vi "Read Address_modified.vi"(0 "VISA resource name":refnum<visa-resource-name>, 5 "Motor ID (0)":u8, 7 "Address number (0)":u8 max=49, 9 "Number of Addresses to read (1)":u8=1, 11 "Error in (no error)":errorcluster) -> (4 "VISA resource name Out":refnum<visa-resource-name>, 6 "Data Read":u8[](array[numeric]), 10 "Motor Error Status":T1, 15 "error out":errorcluster)   [LabVIEW 2015, in "Dynamixel Motor.lvlib"]
doc: "Reads an arbitrary number of consecutive addresses from a motor's register. This is a Low-Level VI that is used by other VIs."
uses:
  <instrlib>/Dynamixel Motor/Public/Motor Operation/Low Level/Alarm Setting.ctl
  <instrlib>/Dynamixel Motor/Dynamixel Motor.lvlib
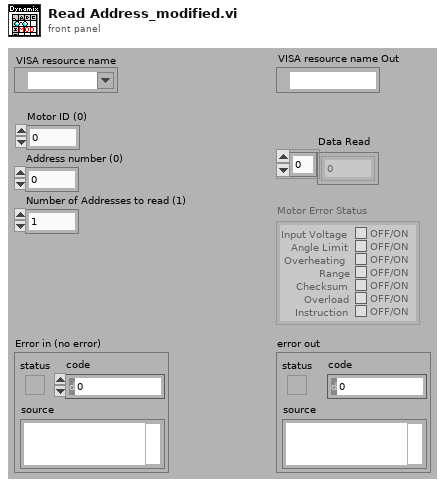
[diagram p1: front panel]
types:
  T1 = typedef "Dynamixel Motor.lvlib/Alarm Setting.ctl" = cluster{"Input Voltage":bool, "Angle Limit":bool, "Overheating ":bool, "Range":bool, "Checksum":bool, "Overload":bool, "Instruction":bool}
  T2 = cluster{"Boolean array[0]":bool, "Boolean array[1]":bool, "Boolean array[2]":bool, "Boolean array[3]":bool, "Boolean array[4]":bool, "Boolean array[5]":bool, "Boolean array[6]":bool}
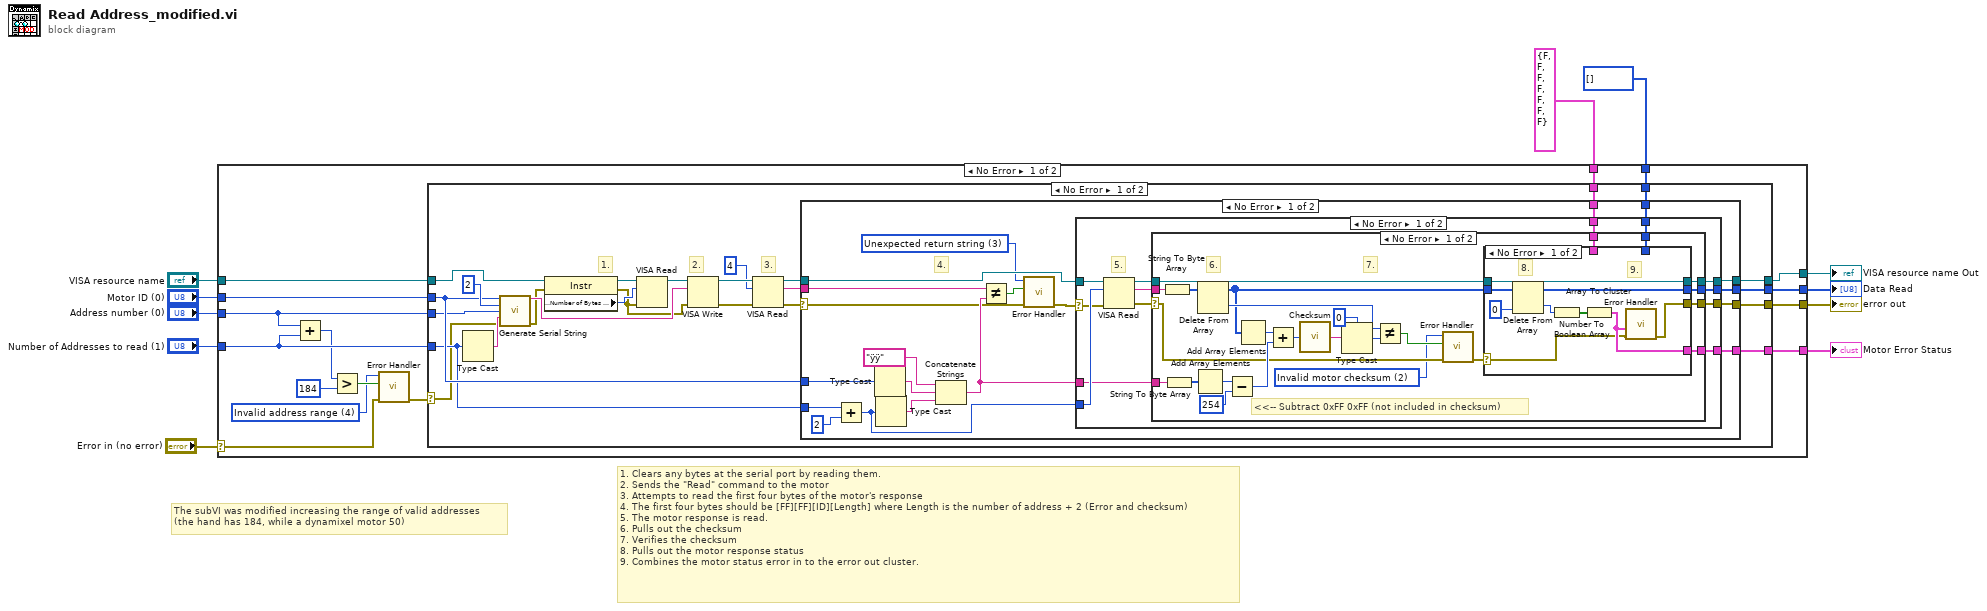
[diagram p0: block diagram]
diagram:
  # "The subVI was modified increasing the range of valid addresses\n(the hand has 184, while a dynamixel motor 50)"
  # "1. Clears any bytes at the serial port by reading them.\n2. Sends the \"Read\" command to the motor\n3. Attempts to read the first four bytes of the motor's response\n4. The first four bytes should be [FF][FF][ID][Length] where Length is the number of address + 2 (Error and checksum)\n5. The motor response is read.\n6. Pulls out the checksum\n7. Verifies the checksum\n8. Pulls out the motor response status\n9. Combines the motor status error in to the error out cluster."
  n1 = case shown="No Error" "Error in (no error)" {
    selector: "Error in (no error)" -> [w16 w143]
    tunnel: "Address number (0)" -> [w20 _]
    tunnel: [w23 w141] -> w10
    tunnel: "VISA resource name" -> [w27 w142]
    tunnel: "Number of Addresses to read (1)" -> [w21 _]
    tunnel: "Motor ID (0)" -> [w25 _]
    tunnel: [w26 w142] -> w6
    tunnel: [w24 w143] -> w5
    tunnel: [w22 w140] -> w3
    tunnel: u8[] [] ("unsigned byte array") -> [w14 w141]
    tunnel: T2 {"Boolean array[0]"=FALSE, "Boolean array[1]"=FALSE, "Boolean array[2]"=FALSE, "Boolean array[3]"=FALSE, "Boolean array[4]"=FALSE, "Boolean array[5]"=FALSE, "Boolean array[6]"=FALSE} ("Boolean array") -> [w13 w140]
    frame No Error {
      w12 = u16 4 items=["Scan timeout"=1, "Invalid motor checksum"=2, "Unexpected return string"=3, "Invalid address range"=4] ("Error type")
      n2 = Add(x=w20, y=w21) -> (x+y=w19:u8)
      n3 = Greater?(x=w19, y=u8 184) -> (0:w15:bool)
      n4 = call <instrlib>:"Error Handler.vi"("error in (no error)"=w16, "Error? (no error)"=w15, "Error type"=w12) -> ("error out"=w17:errorcluster)  [unwired: 8 in]
      n5 = case shown="No Error" w17 {
        selector: w17 -> [w30 w138]
        tunnel: w27 -> [w49 w139]
        tunnel: [w48 w139] -> w26
        tunnel: w25 -> [w42 _]
        tunnel: [w40 w138] -> w24
        tunnel: [w39 w137] -> w23
        tunnel: [w38 w136] -> w22
        tunnel: w21 -> [w32 _]
        tunnel: w20 -> [w31 _]
        tunnel: w14 -> [w29 w137]
        tunnel: w13 -> [w28 w136]
        frame No Error {
          # "3."
          # "2."
          # "1."
          n6 = Type Cast(x=w32) -> (*(type *) &x=w33:string)  [unwired: 1 in]
          n7 = call <instrlib>:"Generate Serial String.vi"("Motor ID"=w42, "Command"=u8 2, "Address"=w31, "Parameters"=w33, "Error in (no error)"=w30) -> ("Command to Serial"=w50:string, "error out"=w45:errorcluster)  [unwired: 9 in]
          n8 = property class="Instr"(reference=w49, error in=w45) -> (reference out=w46:refnum<visa-resource-name>, error out=w41:errorcluster, "Serial Settings:Number of Bytes at Serial Port"=w47:u32)
          n9 = VISA Read(VISA resource name=w46, byte count=w47, error in (no error)=w41) -> (VISA resource name out=w52:refnum<visa-resource-name>)  [unwired: 3 out]
          n10 = VISA Write(VISA resource name=w52, write buffer=w50, error in (no error)=w41) -> (VISA resource name out=w51:refnum<visa-resource-name>, error out=w44:errorcluster)  [unwired: 1 out]
          n11 = VISA Read(VISA resource name=w51, byte count=u32 4, error in (no error)=w44) -> (VISA resource name out=w34:refnum<visa-resource-name>, read buffer=w37:string, error out=w35:errorcluster)  [unwired: 1 out]
          n12 = case shown="No Error" w35 {
            selector: w35 -> [w58 w135]
            tunnel: w32 -> [w71 _]
            tunnel: w42 -> [w70 _]
            tunnel: w37 -> [w57 _]
            tunnel: [w64 w135] -> w40
            tunnel: w34 -> [w66 w134]
            tunnel: [w65 w134] -> w48
            tunnel: [w61 w133] -> w39
            tunnel: [w60 w132] -> w38
            tunnel: w29 -> [w55 w133]
            tunnel: w28 -> [w54 w132]
            frame No Error {
              w53 = u16 3 items=["Scan timeout"=1, "Invalid motor checksum"=2, "Unexpected return string"=3, "Invalid address range"=4] ("Error type")
              # "4."
              n13 = Add(x=w71, y=u8 2) -> (x+y=w63:u8)
              n14 = Type Cast(x=w70) -> (*(type *) &x=w69:string)  [unwired: 1 in]
              n15 = Type Cast(x=w63) -> (*(type *) &x=w68:string)  [unwired: 1 in]
              n16 = Concatenate Strings("ÿÿ" ("string"), w69, w68) -> (w62:string)
              n17 = Not Equal?(x=w57, y=w62) -> (x != y?=w56:bool)
              n18 = call <instrlib>:"Error Handler.vi"("error in (no error)"=w58, "Error? (no error)"=w56, "Error type"=w53) -> ("error out"=w59:errorcluster)  [unwired: 8 in]
              n19 = case shown="No Error" w59 {
                selector: w59 -> [w75 w130]
                tunnel: w66 -> [w85 w131]
                tunnel: [w77 w131] -> w65
                tunnel: [w81 w130] -> w64
                tunnel: w63 -> [w84 _]
                tunnel: w62 -> [w80 _]
                tunnel: [w79 w129] -> w61
                tunnel: [w78 w128] -> w60
                tunnel: w55 -> [w74 w129]
                tunnel: w54 -> [w73 w128]
                frame No Error {
                  # "5."
                  n20 = VISA Read(VISA resource name=w85, byte count=w84, error in (no error)=w75) -> (VISA resource name out=w76:refnum<visa-resource-name>, read buffer=w83:string, error out=w82:errorcluster)  [unwired: 1 out]
                  n21 = case shown="No Error" w82 {
                    selector: w82 -> [w91 w127]
                    tunnel: w83 -> [w96 _]
                    tunnel: [w101 w127] -> w81
                    tunnel: w80 -> [w110 _]
                    tunnel: [w100 w125] -> w79
                    tunnel: [w92 w124] -> w78
                    tunnel: [w95 w126] -> w77
                    tunnel: w76 -> [w94 w126]
                    tunnel: w74 -> [w88 w125]
                    tunnel: w73 -> [w87 w124]
                    frame No Error {
                      w86 = u16 2 items=["Scan timeout"=1, "Invalid motor checksum"=2, "Unexpected return string"=3, "Invalid address range"=4] ("Error type")
                      # "<<-- Subtract 0xFF 0xFF (not included in checksum)"
                      # "7."
                      # "6."
                      n22 = String To Byte Array(string=w96) -> (unsigned byte array=w93:u8[])
                      n23 = String To Byte Array(string=w110) -> (unsigned byte array=w109:u8[])
                      n24 = Add Array Elements(numeric array=w109) -> (sum=w99:u8)
                      n25 = Delete From Array(array=w93) -> (deleted portion=w103:u8, array with subset deleted=w102:u8[])  [unwired: 2 in]
                      n26 = Subtract(x=w99, y=u8 254) -> (x-y=w97:u8)
                      n27 = Add Array Elements(numeric array=w102) -> (sum=w106:u8)
                      n28 = Add(x=w106, y=w97) -> (x+y=w105:u8)
                      n29 = call <instrlib>:"Checksum.vi"("Sum of bytes"=w105) -> ("Checksum String"=w108:string)
                      n30 = Type Cast(type=u8 0, x=w108) -> (*(type *) &x=w104:u8)
                      n31 = Not Equal?(x=w103, y=w104) -> (x != y?=w89:bool)
                      n32 = call <instrlib>:"Error Handler.vi"("error in (no error)"=w91, "Error? (no error)"=w89, "Error type"=w86) -> ("error out"=w90:errorcluster)  [unwired: 8 in]
                      n33 = case shown="No Error" w90 {
                        selector: w90 -> [w111 w122]
                        tunnel: [w117 w121] -> w100
                        tunnel: w102 -> [w118 _]
                        tunnel: [w112 w122] -> w101
                        tunnel: [w119 w123] -> w95
                        tunnel: w94 -> [w119 w123]
                        tunnel: [w113 w120] -> w92
                        tunnel: w88 -> [_ w121]
                        tunnel: w87 -> [_ w120]
                        frame No Error {
                          # "8."
                          # "9."
                          n34 = Delete From Array(array=w118, index=0) -> (deleted portion=w114:u8, array with subset deleted=w117:u8[])  [unwired: 1 in]
                          n35 = Number To Boolean Array(number=w114) -> (Boolean array=w115:bool[])
                          n36 = Array To Cluster(array=w115) -> (cluster=w113:T2)
                          n37 = call <instrlib>:"Error Handler.vi"("error in (no error)"=w111, "Motor Error Status (none)"=w113) -> ("error out"=w112:errorcluster)  [unwired: 9 in]
                        }
                        frame Error {
                        }
                      }
                    }
                    frame Error {
                    }
                  }
                }
                frame Error {
                }
              }
            }
            frame Error {
            }
          }
        }
        frame Error {
        }
      }
    }
    frame Error {
    }
  }
  "Data Read" <- w10
  "VISA resource name Out" <- w6
  "error out" <- w5
  "Motor Error Status" <- w3
